vi "AthenaXbox.vi"() -> (2 "R Thumb":i32(slide) scale=-32768.0..32768.0)   [LabVIEW 2009]
uses:
  <vilib>/Utility/inputDevices.llb/closeJoystick.vi
  <vilib>/Utility/inputDevices.llb/joystickAcquire.vi
  <vilib>/Utility/Variable/NI_VariableUtilities.lvlib
panel:
  out "mouse info":T1(array[cluster])
  out "key info":T2(array[cluster])
  in  "device index":i32
  in  "ms/refresh":u32=20
  in  "Stop":bool
  out "Start":bool
  out "Stop/Back":bool
  out "Right trigger":bool
  out "Left Trigger":bool
  out "Cluster":T3
  out "LThumb":i32(slide) scale=-32768.0..32768.0
  out "Left Thumb button":bool
  out "Right Thumb button":bool
  out "LB":bool
  out "RB":bool
  out "Y":bool
  out "X":bool
  out "B":bool
  out "A":bool caption="Boolean"
  out "Joystick Info":T4(array[cluster])
  out "Direction Info":T5
  out "Button Info":T6
  out "Axis Info":T7
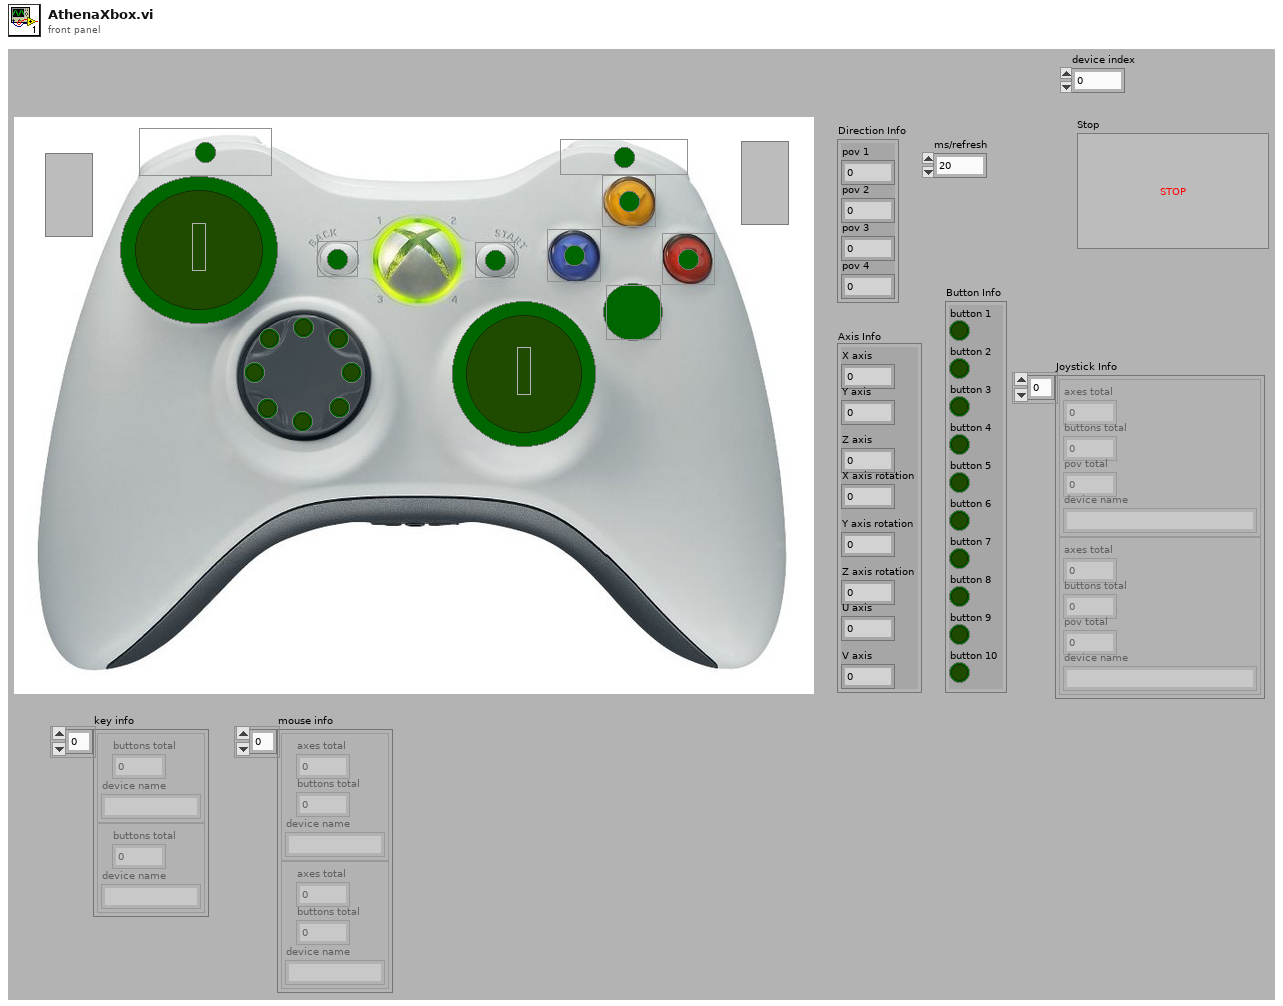
[diagram p1: front panel]
types:
  T1 = cluster{"axes total":u32, "buttons total":u32, "device name":string}[]
  T2 = cluster{"buttons total":u32, "device name":string}[]
  T3 = cluster{"Boolean 4":bool, "Boolean 6":bool, "Boolean 3":bool, "Boolean 7":bool, "Boolean 2":bool, "Boolean 9":bool, "Boolean 5":bool, "Boolean 8":bool}
  T4 = cluster{"axes total":u32, "buttons total":u32, "pov total":u32, "device name":string}[]
  T5 = cluster{"pov 1":i32, "pov 2":i32, "pov 3":i32, "pov 4":i32}
  T6 = cluster{"button 1":bool, "button 2":bool, "button 3":bool, "button 4":bool, "button 5":bool, "button 6":bool, "button 7":bool, "button 8":bool, "button 9":bool, "button 10":bool, "button 11":bool, "button 12":bool, "button 13":bool, "button 14":bool, "button 15":bool, "button 16":bool, "button 17":bool, "button 18":bool, "button 19":bool, "button 20":bool, "button 21":bool, "button 22":bool, "button 23":bool, "button 24":bool, "button 25":bool, "button 26":bool, "button 27":bool, "button 28":bool, "button 29":bool, "button 30":bool, "button 31":bool, "button 32":bool}
  T7 = cluster{"X axis":i32, "Y axis":i32, "Z axis":i32, "X axis rotation":i32, "Y axis rotation":i32, "Z axis rotation":i32, "U axis":i32, "V axis":i32}
  T8 = cluster{"Array[0]":bool, "Array[1]":bool, "Array[2]":bool, "Array[3]":bool, "Array[4]":bool, "Array[5]":bool, "Array[6]":bool, "Array[7]":bool}
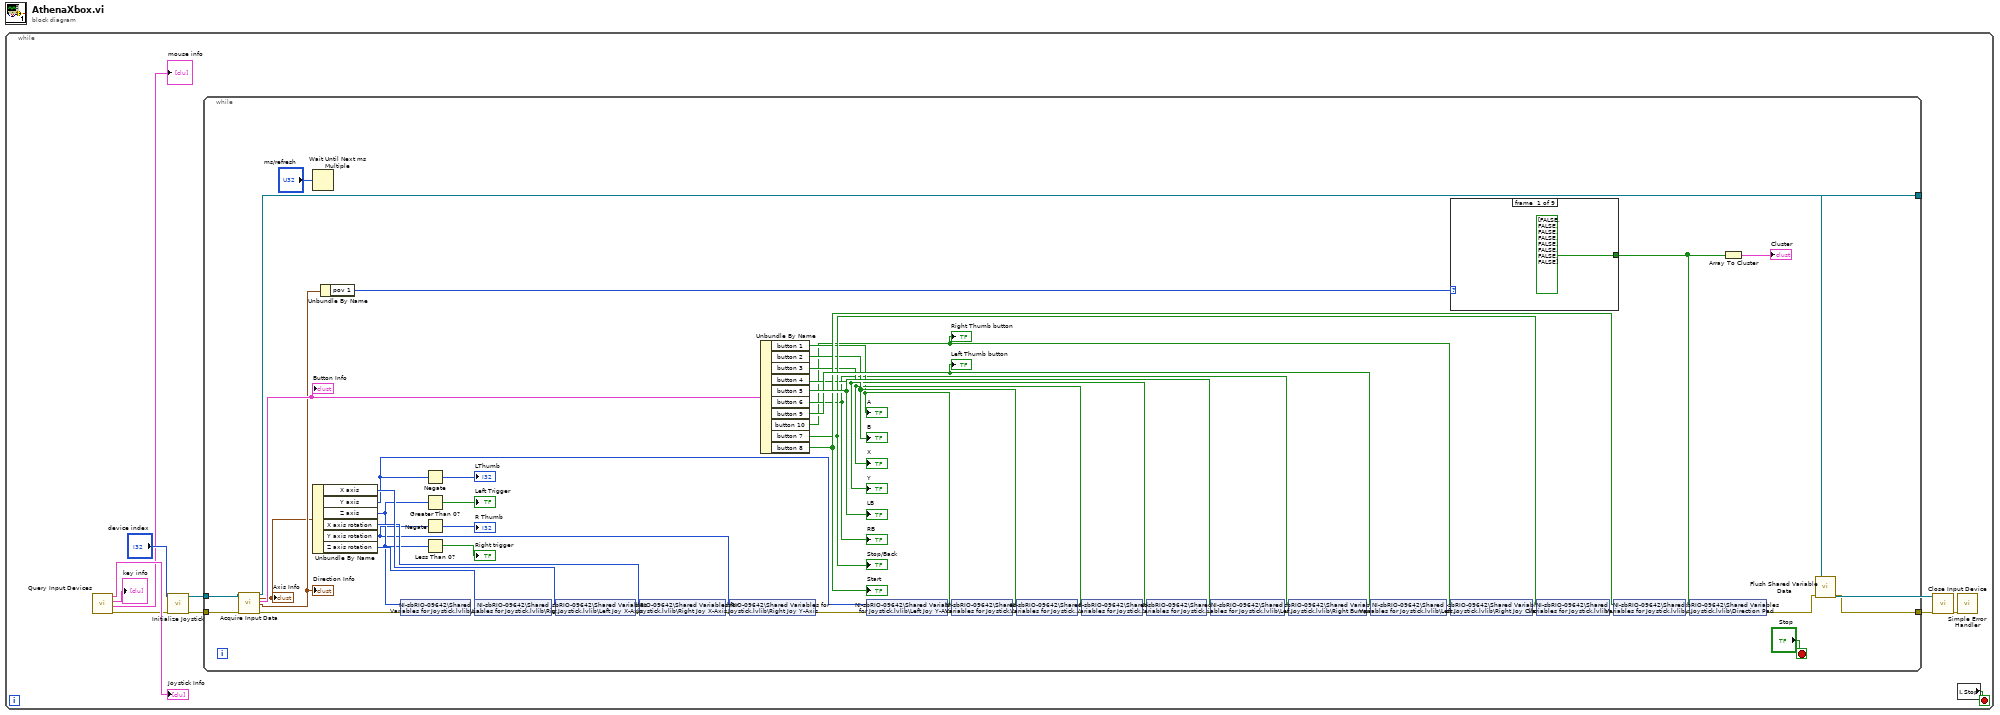
[diagram p0: block diagram]
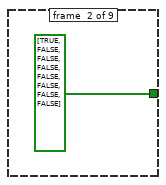
[diagram p2: hidden frame]
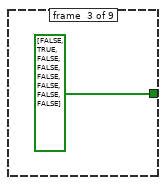
[diagram p3: hidden frame]
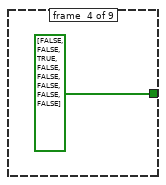
[diagram p4: hidden frame]
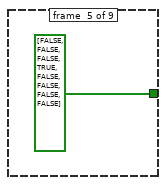
[diagram p5: hidden frame]
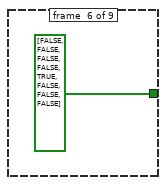
[diagram p6: hidden frame]
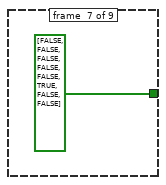
[diagram p7: hidden frame]
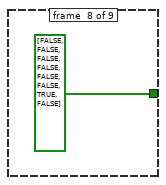
[diagram p8: hidden frame]
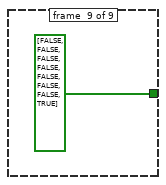
[diagram p9: hidden frame]
diagram:
  n1 = while {
    stop <- w3 stop-if-true
    n2 = call <vilib>:"Query Input Devices.vi"() -> ("error out"=w5:errorcluster, "mouse info"=→"mouse info":T1, "key info"=→"key info":T2, "joystick info"=→"Joystick Info":T4)  [unwired: 1 in, 7 out]
    n3 = call <vilib>:"Initialize Joystick.vi"("error in (no error)"=w5, "device index"="device index") -> ("error out"=w9:errorcluster, "device ID"=w10:refnum<k1>)  [unwired: 8 out]
    n4 = while {
      tunnel: w10 -> [w61]
      tunnel: w9 -> [w60]
      tunnel: [w59] -> w8
      tunnel: [w12] -> w7
      stop <- "Stop" stop-if-true
      n5 = call-poly <vilib>:"Acquire Input Data.vi"("device ID"=w61, "error in (no error)"=w60) -> ("device ID"=w59:refnum<k1>, "axis info"=w51:T7, "button info"=w58:T6, "direction info"=w57:T5, "error out"=w14:errorcluster)  [unwired: 13 out]
      "Axis Info" <- w51
      "Button Info" <- w58
      "Direction Info" <- w57
      n6 = Wait Until Next ms Multiple(millisecond multiple="ms/refresh") -> ()  [unwired: 1 out]
      n7 = Unbundle By Name(w51) -> ("X axis"=w22:i32, "Y axis"=w20:i32, "Z axis"=w18:i32, "X axis rotation"=w21:i32, "Y axis rotation"=w17:i32, "Z axis rotation"=w19:i32)
      n8 = Unbundle By Name(w57) -> ("pov 1"=w56:i32)
      n9 = shared-variable "NI-sbRIO-09642\\Shared Variables for Joystick.lvlib\\Left Trigger"(w18, error in=w14) -> (error out=w37:errorcluster)
      n10 = Negate(x=w20) -> (-x=→"LThumb":i32)
      n11 = Greater Than 0?(x=w18) -> (x > 0?=→"Left Trigger":bool)
      n12 = Negate(x=w17) -> (-x=→"R Thumb":i32)
      n13 = Less Than 0?(x=w18) -> (x < 0?=→"Right trigger":bool)
      n14 = shared-variable "NI-sbRIO-09642\\Shared Variables for Joystick.lvlib\\Right Trigger"(w19, error in=w37) -> (error out=w23:errorcluster)
      n15 = shared-variable "NI-sbRIO-09642\\Shared Variables for Joystick.lvlib\\Left Joy X-Axis"(w22, error in=w23) -> (error out=w24:errorcluster)
      n16 = shared-variable "NI-sbRIO-09642\\Shared Variables for Joystick.lvlib\\Right Joy X-Axis"(w21, error in=w24) -> (error out=w15:errorcluster)
      n17 = shared-variable "NI-sbRIO-09642\\Shared Variables for Joystick.lvlib\\Right Joy Y-Axis"(w17, error in=w15) -> (error out=w16:errorcluster)
      n18 = Unbundle By Name(w58) -> ("button 1"=w40:bool, "button 2"=w43:bool, "button 3"=w41:bool, "button 4"=w42:bool, "button 5"=w50:bool, "button 6"=w39:bool, "button 9"=w49:bool, "button 10"=w38:bool, "button 7"=w45:bool, "button 8"=w46:bool)
      "A" <- w40
      "B" <- w43
      "Y" <- w42
      "X" <- w41
      "RB" <- w39
      "LB" <- w50
      "Left Thumb button" <- w49
      "Right Thumb button" <- w38
      "Stop/Back" <- w45
      "Start" <- w46
      n19 = shared-variable "NI-sbRIO-09642\\Shared Variables for Joystick.lvlib\\Left Joy Y-Axis"(w20, error in=w16) -> (error out=w25:errorcluster)
      n20 = shared-variable "NI-sbRIO-09642\\Shared Variables for Joystick.lvlib\\A Button"(w40, error in=w25) -> (error out=w26:errorcluster)
      n21 = shared-variable "NI-sbRIO-09642\\Shared Variables for Joystick.lvlib\\B Button"(w43, error in=w26) -> (error out=w27:errorcluster)
      n22 = shared-variable "NI-sbRIO-09642\\Shared Variables for Joystick.lvlib\\X Button"(w41, error in=w27) -> (error out=w28:errorcluster)
      n23 = shared-variable "NI-sbRIO-09642\\Shared Variables for Joystick.lvlib\\Y Button"(w42, error in=w28) -> (error out=w29:errorcluster)
      n24 = shared-variable "NI-sbRIO-09642\\Shared Variables for Joystick.lvlib\\Left Bumper"(w50, error in=w29) -> (error out=w30:errorcluster)
      n25 = shared-variable "NI-sbRIO-09642\\Shared Variables for Joystick.lvlib\\Right Bumper"(w39, error in=w30) -> (error out=w31:errorcluster)
      n26 = shared-variable "NI-sbRIO-09642\\Shared Variables for Joystick.lvlib\\Left Joy Click"(w49, error in=w31) -> (error out=w32:errorcluster)
      n27 = case shown="-1, Default" w56 {
        tunnel: [bool[] [FALSE, FALSE, FALSE, FALSE, FALSE, FALSE, FALSE, FALSE] ("Array") bool[] [TRUE, FALSE, FALSE, FALSE, FALSE, FALSE, FALSE, FALSE] ("Array") bool[] [FALSE, TRUE, FALSE, FALSE, FALSE, FALSE, FALSE, FALSE] ("Array") bool[] [FALSE, FALSE, TRUE, FALSE, FALSE, FALSE, FALSE, FALSE] ("Array") bool[] [FALSE, FALSE, FALSE, TRUE, FALSE, FALSE, FALSE, FALSE] ("Array") bool[] [FALSE, FALSE, FALSE, FALSE, TRUE, FALSE, FALSE, FALSE] ("Array") bool[] [FALSE, FALSE, FALSE, FALSE, FALSE, TRUE, FALSE, FALSE] ("Array") bool[] [FALSE, FALSE, FALSE, FALSE, FALSE, FALSE, TRUE, FALSE] ("Array") bool[] [FALSE, FALSE, FALSE, FALSE, FALSE, FALSE, FALSE, TRUE] ("Array")] -> w36
        frame #0 {
        }
        frame #1 {
        }
        frame #2 {
        }
        frame #3 {
        }
        frame #4 {
        }
        frame #5 {
        }
        frame #6 {
        }
        frame #7 {
        }
        frame #8 {
        }
      }
      n28 = shared-variable "NI-sbRIO-09642\\Shared Variables for Joystick.lvlib\\Right Joy Click"(w38, error in=w32) -> (error out=w33:errorcluster)
      n29 = shared-variable "NI-sbRIO-09642\\Shared Variables for Joystick.lvlib\\Back Button"(w45, error in=w33) -> (error out=w35:errorcluster)
      n30 = shared-variable "NI-sbRIO-09642\\Shared Variables for Joystick.lvlib\\Start Button"(w46, error in=w35) -> (error out=w34:errorcluster)
      n31 = shared-variable "NI-sbRIO-09642\\Shared Variables for Joystick.lvlib\\Direction Pad"(w36, error in=w34) -> (error out=w13:errorcluster)
      n32 = Array To Cluster(array=w36) -> (cluster=→"Cluster":T8)
      n33 = call <vilib>:"Flush Shared Variable Data.vi"("error in (no error)"=w13) -> ("error out"=w12:errorcluster)  [unwired: 10 in]
    }
    n34 = call-poly <vilib>:"Close Input Device.vi"("error in (no error)"=w7, "device ID"=w8) -> ("error out"=w4:errorcluster)  [unwired: 8 out]
    n35 = call <vilib>:"Simple Error Handler.vi"("error in (no error)"=w4) -> ()  [unwired: 1 in, 8 out]
    n36 = local read "Stop"() -> (w3:bool)
  }
